vi "2Gear.vi"(8 "error in":errorcluster, 10 "2 Gear Side":enum16{"Left", "Right"}(ring), 11 "Gear Side":enum16{"Center", "Left", "Right"}(ring)) -> (0 "error out":errorcluster)   [LabVIEW 2016]
doc: "Robot picks up a second gear and scores it on the peg"
uses:
  Robot Global Data.vi
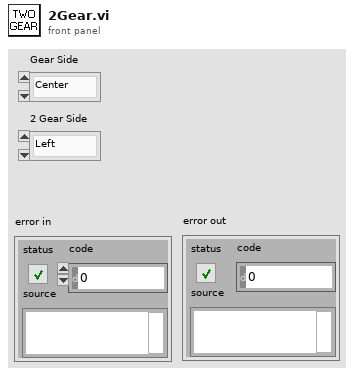
[diagram p1: front panel]
types:
  T1 = cluster{"CenterBack":dbl, "CenterTurn":dbl, "SideBack":dbl, "SideTurn":dbl, "ScanSpeed":dbl, "IntakeSpeed":dbl, "StopDist":dbl, "Config":cluster{"Lower X":dbl, "Lower Y":dbl, "Upper X":dbl, "Upper Y":dbl}}
  T2 = cluster{"ArmDist":dbl, "StopDist":dbl, "Config":cluster{"Lower X":dbl, "Lower Y":dbl, "Upper X":dbl, "Upper Y":dbl}, "WiggleAmount":dbl, "WigglePeriod":u32, "ForwardAmount":dbl, "ForwardTime":u32, "BackSpeed":dbl, "BackTime":u32}
  T3 = cluster{"Target?":bool, "Angle":dbl, "Distance":dbl, "NewAngle":dbl}
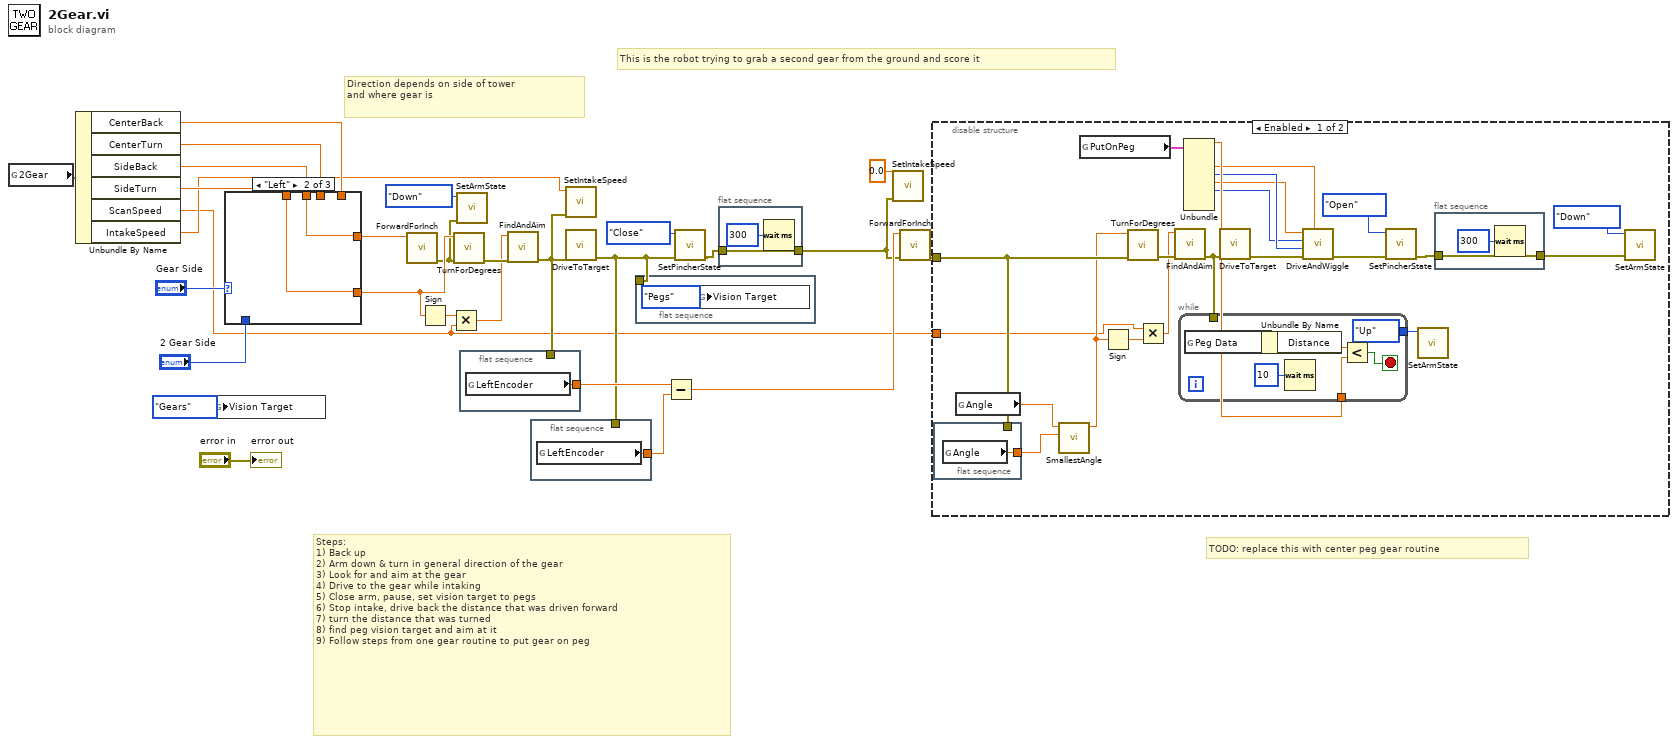
[diagram p0: block diagram]
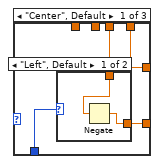
[diagram p3: hidden frame]
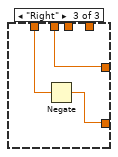
[diagram p5: hidden frame]
diagram:
  # "TODO: replace this with center peg gear routine"
  # "Direction depends on side of tower\nand where gear is"
  # "Steps:\n1) Back up\n2) Arm down & turn in general direction of the gear\n3) Look for and aim at the gear\n4) Drive to the gear while intaking\n5) Close arm, pause, set vision target to pegs\n6) Stop intake, drive back the distance that was driven forward\n7) turn the distance that was turned\n8) find peg vision target and aim at it\n9) Follow steps from one gear routine to put gear on peg"
  # "This is the robot trying to grab a second gear from the ground and score it"
  n1 = global read "Robot Global Data.vi" "2Gear"() -> (w7:T1)
  n2 = Unbundle By Name(w7) -> ("CenterBack"=w6:dbl, "CenterTurn"=w5:dbl, "SideBack"=w4:dbl, "SideTurn"=w3:dbl, "ScanSpeed"=w1:dbl, "IntakeSpeed"=w2:dbl)
  n3 = global write "Robot Global Data.vi" "Vision Target"(enum16{"Pegs", "Gears"}."Gears" ("Vision Target")) -> ()
  n4 = case shown="\"Left\"" "Gear Side" {
    tunnel: "2 Gear Side" -> [w32 _ _]
    tunnel: [w31 w36 w38] -> w23
    tunnel: [w30 w37 w40] -> w25
    tunnel: w6 -> [w30 _ _]
    tunnel: w5 -> [w29 _ _]
    tunnel: w4 -> [_ w37 w40]
    tunnel: w3 -> [_ w36 w39]
    frame "Center", Default {
      n5 = case shown="\"Left\", Default" w32 {
        tunnel: [w34 w35] -> w31
        tunnel: w29 -> [w33 w35]
        frame "Left", Default {
          n6 = Negate(x=w33) -> (-x=w34:dbl)
        }
        frame "Right" {
        }
      }
    }
    frame "Left" {
    }
    frame "Right" {
      n7 = Negate(x=w39) -> (-x=w38:dbl)
    }
  }
  n8 = call "ForwardForInch.vi"("Distance"=w25) -> ("error out"=w15:errorcluster)  [unwired: 10 in]
  n9 = Sign(1:w23) -> (0:w22:dbl)
  n10 = Multiply(x=w22, y=w1) -> (x*y=w21:dbl)
  n11 = call "TurnForDegrees.vi"("error in"=w15, "Angle"=w23) -> ("error out"=w24:errorcluster)  [unwired: 9 in]
  n12 = call "SetArmState.vi"("error in"=w15, "ArmState"=enum16{"Up", "Down"}."Down") -> ()  [unwired: 9 in, 1 out]
  n13 = flat-sequence {
    tunnel: w13 -> [_]
    tunnel: [w41] -> w19
    frame #0 {
      n14 = global read "Robot Global Data.vi" "LeftEncoder"() -> (w41:dbl)
    }
  }
  n15 = call "FindAndAim.vi"("error in"=w24, "Speed/Direction"=w21) -> ("error out"=w13:errorcluster)  [unwired: 9 in]
  n16 = flat-sequence {
    tunnel: [w42] -> w18
    tunnel: w11 -> [_]
    frame #0 {
      n17 = global read "Robot Global Data.vi" "LeftEncoder"() -> (w42:dbl)
    }
  }
  n18 = call "SetIntakeSpeed.vi"("error in"=w13, "Speed"=w2) -> ()  [unwired: 9 in, 1 out]
  n19 = call "DriveToTarget.vi"("error in"=w13) -> ("error out"=w11:errorcluster)  [unwired: 10 in]
  n20 = flat-sequence {
    tunnel: w11 -> [_]
    frame #0 {
      n21 = global write "Robot Global Data.vi" "Vision Target"(enum16{"Pegs", "Gears"}."Pegs" ("Vision Target")) -> ()
    }
  }
  n22 = Subtract(x=w19, y=w18) -> (x-y=w17:dbl)
  n23 = call "SetPincherState.vi"("error in"=w11, "PincherState"=enum16{"Open", "Close"}."Close") -> ("error out"=w9:errorcluster)  [unwired: 9 in]
  n24 = flat-sequence {
    tunnel: w9 -> [w44]
    tunnel: [w44] -> w8
    frame #0 {
      n25 = Wait (ms)(milliseconds to wait=u32 300) -> ()  [unwired: 1 out]
    }
  }
  n26 = call "SetIntakeSpeed.vi"("error in"=w8, "Speed"=0.0) -> ()  [unwired: 9 in, 1 out]
  n27 = call "ForwardForInch.vi"("error in"=w8, "Distance"=w17) -> ("error out"=w16:errorcluster)  [unwired: 9 in]
  n28 = disable-structure shown="Enabled" {
    disable-tunnel: w16 -> [w66 _]
    disable-tunnel: w1 -> [w53 _]
    frame Enabled {
      n29 = flat-sequence {
        tunnel: [w76] -> w62
        tunnel: w66 -> [_]
        frame #0 {
          n30 = global read "Robot Global Data.vi" "Angle"() -> (w76:dbl)
        }
      }
      n31 = global read "Robot Global Data.vi" "Angle"() -> (w61:dbl)
      n32 = call "SmallestAngle.vi"("Angle B"=w62, "Angle A"=w61) -> ("Smallest B to A"=w63:dbl)  [unwired: 9 in]
      n33 = global read "Robot Global Data.vi" "PutOnPeg"() -> (w52:T2)
      n34 = Sign(1:w63) -> (0:w65:dbl)
      n35 = call "TurnForDegrees.vi"("error in"=w66, "Angle"=w63) -> ("error out"=w67:errorcluster)  [unwired: 9 in]
      n36 = Multiply(x=w53, y=w65) -> (x*y=w64:dbl)
      n37 = call "FindAndAim.vi"("error in"=w67, "Speed/Direction"=w64) -> ("error out"=w58:errorcluster)  [unwired: 9 in]
      n38 = Unbundle(w52) -> ("ArmDist"=w51:dbl, "WiggleAmount"=w49:dbl, "WigglePeriod"=w48:u32, "ForwardAmount"=w46:dbl, "ForwardTime"=w47:u32)  [unwired: 4 out]
      n39 = while {
        tunnel: [enum16{"Up", "Down"}."Up" ("ArmState")] -> w59
        tunnel: w58 -> [_]
        tunnel: w51 -> [w71]
        stop <- w73 stop-if-true
        n40 = global read "Robot Global Data.vi" "Peg Data"() -> (w75:T3)
        n41 = Unbundle By Name(w75) -> ("Distance"=w74:dbl)
        n42 = Wait (ms)(milliseconds to wait=u32 10) -> ()  [unwired: 1 out]
        n43 = Less?(x=w74, y=w71) -> (x < y?=w73:bool)
      }
      n44 = call "DriveToTarget.vi"("error in"=w58) -> ("error out"=w50:errorcluster)  [unwired: 10 in]
      n45 = call "DriveAndWiggle.vi"("Wiggle amount"=w49, "error in"=w50, "Wiggle Period (ms)"=w48, "Time (ms)"=w47, "Speed/Direction"=w46) -> ("error out"=w57:errorcluster)  [unwired: 6 in]
      n46 = call "SetPincherState.vi"("error in"=w57, "PincherState"=enum16{"Open", "Close"}."Open") -> ("error out"=w56:errorcluster)  [unwired: 9 in]
      n47 = call "SetArmState.vi"("ArmState"=w59) -> ()  [unwired: 10 in, 1 out]
      n48 = flat-sequence {
        tunnel: w56 -> [w68]
        tunnel: [w68] -> w54
        frame #0 {
          n49 = Wait (ms)(milliseconds to wait=u32 300) -> ()  [unwired: 1 out]
        }
      }
      n50 = call "SetArmState.vi"("error in"=w54, "ArmState"=enum16{"Up", "Down"}."Down") -> ()  [unwired: 9 in, 1 out]
    }
    frame Disabled {
    }
  }
  "error out" <- "error in"
